vi "gds_usrp_tx.vi"() -> ()   [LabVIEW 2012]
uses:
  <instrlib>/niUSRP/niUSRP Write Tx Data (CDB Cluster).vi
  <vilib>/addons/Modulation/niDMT.lvlib
panel:
  in  "stop":bool
  out "Key Bit Sequence":i8[](array[numeric])
  in  "Plots":enum32{"Constellation", "Transmitted Signal"}(tab)
  out "Constellation Graph":T1(graph) caption="Transmitted Constellation Graph"
  out "Transmitted I Waveform Graph":waveform(dbl)(graph)
  out "Transmitted Q  Waveform Graph":waveform(dbl)(graph)
  out "coerced gain":dbl format="%#_6f"
  out "coerced carrier frequency":dbl=100000.0 format="%#_6p"
  out "coerced IQ rate":dbl=100000.0 format="%#_6p"
  in  "gain":dbl=20.0 format="%#_6f"
  in  "carrier frequency":dbl=433001000.0 format="%#_6p"
  in  "active antenna":string="TX1"
  in  "device names":refnum<k15>="192.168.10.26"
  out "error out":errorcluster
  in  "Modulation Parameters":T2={"TX Parameters"={"Sampling Rate"=1000000.0, "Oversample Factor"=2}, "Shared Parameters"={"Packet Length"=500, "Preamble Length"=20, "modulation type"=enum."OOK", "FSK deviation (Hz)"=625.0, "Filter Parameters"={"modulation type"=enum."ASK", "pulse shaping filter (none)"=enum."none", "filter length (symbols)"=8, "filter parameter"=0.5}}}
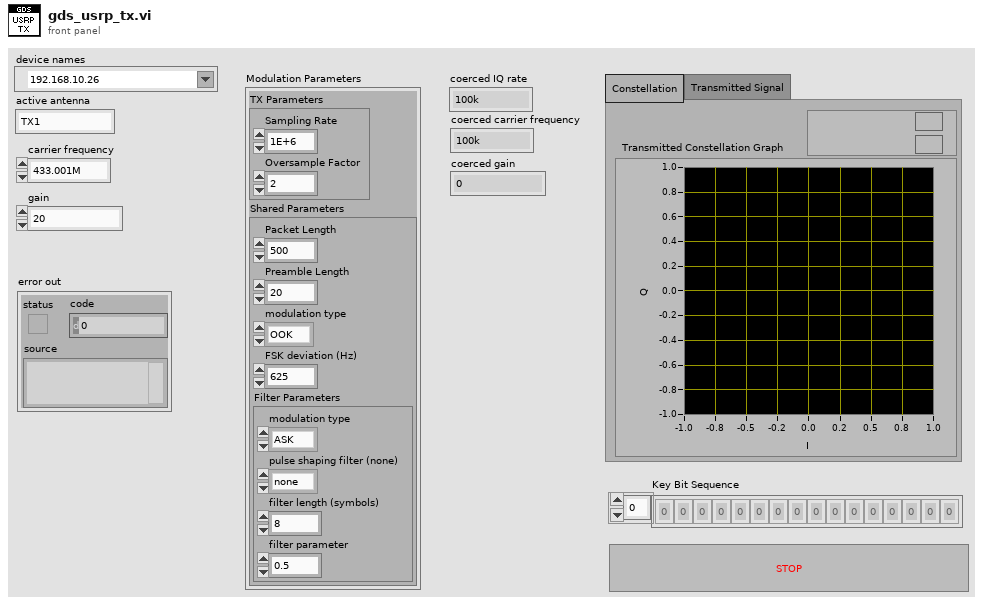
[diagram p1: front panel]
types:
  T1 = cluster{"Decimated Array":dbl[], "Decimated Array":dbl[]}[]
  T2 = cluster{"TX Parameters":cluster{"Sampling Rate":dbl, "Oversample Factor":i32}, "Shared Parameters":cluster{"Packet Length":i32, "Preamble Length":i32, "modulation type":enum16{"OOK", "FSK", "PSK", "QAM", "MSK", "PAM", "ASK", "CPM"}, "FSK deviation (Hz)":dbl, "Filter Parameters":cluster{"modulation type":enum16{"FSK", "PSK", "QAM", "MSK", "PAM", "ASK", "CPM"}, "pulse shaping filter (none)":enum16{"none", "Raised Cosine", "Root Raised Cos", "Gaussian"}, "filter length (symbols)":i32, "filter parameter":dbl}}}
  T3 = typedef "niAMT.lvlib/Complex Data Waveform.ctl" = cluster{"t0":dbl, "dt":dbl, "Y":cdb[]}
  T4 = cluster{"constellation":dbl[], "oversampled data":dbl[]}[]
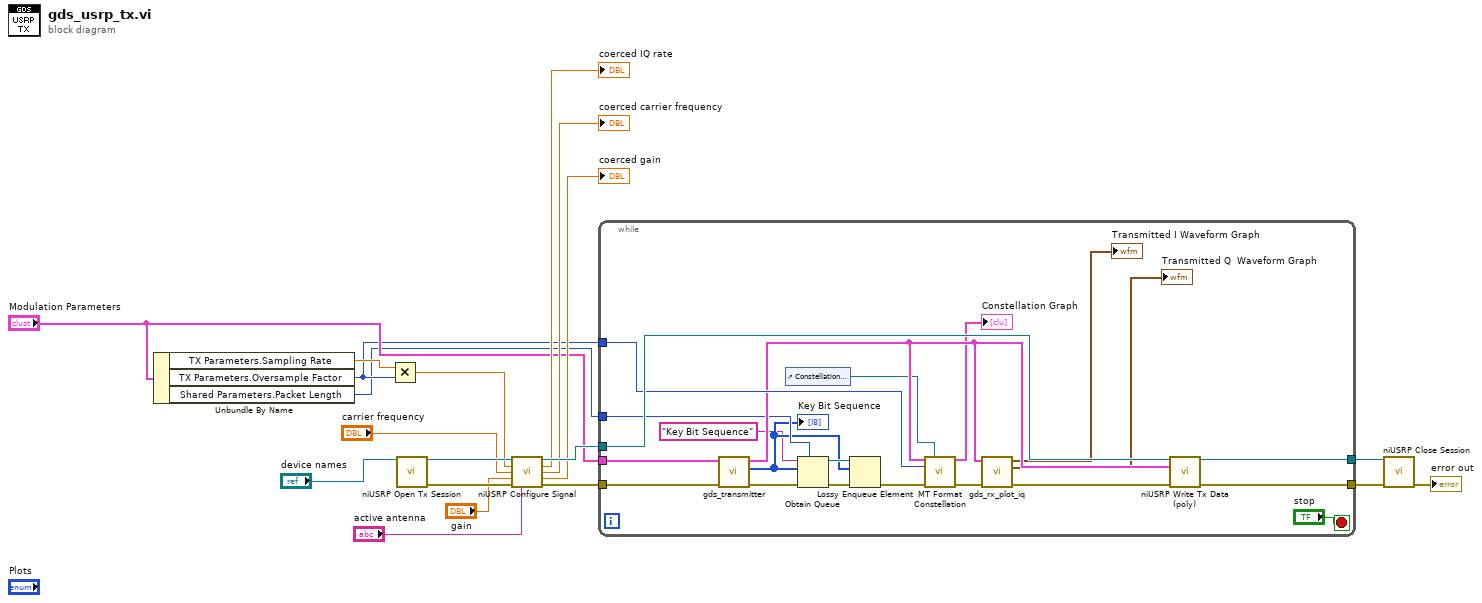
[diagram p0: block diagram]
diagram:
  n1 = Unbundle By Name("Modulation Parameters") -> ("TX Parameters.Sampling Rate"=w4:dbl, "TX Parameters.Oversample Factor"=w2:i32, "Shared Parameters.Packet Length"=w1:i32)
  n2 = Multiply(x=w4, y=w2) -> (x*y=w3:dbl)
  n3 = call <instrlib>:"niUSRP Open Tx Session.vi"("device names"="device names") -> ("session handle out"=w18:refnum<k15>, "error out"=w19:errorcluster)  [unwired: 13 in]
  n4 = call <instrlib>:"niUSRP Configure Signal.vi"("session handle"=w18, "IQ rate"=w3, "carrier frequency"="carrier frequency", "gain"="gain", "error in (no error)"=w19, "active antenna"="active antenna") -> ("session handle out"=w17:refnum<k15>, "coerced IQ rate"=→"coerced IQ rate":dbl, "coerced carrier frequency"=→"coerced carrier frequency":dbl, "coerced gain"=→"coerced gain":dbl, "error out"=w14:errorcluster)  [unwired: 5 in]
  n5 = while {
    tunnel: w17 -> [w40]
    tunnel: [w39] -> w16
    tunnel: [w38] -> w15
    tunnel: w14 -> [w37]
    tunnel: "Modulation Parameters" -> [w36]
    tunnel: w2 -> [w35]
    tunnel: w1 -> [w30]
    stop <- "stop" stop-if-true
    n6 = call "gds_transmitter.vi"("error in (no error)"=w37, "Modulation Parameters"=w36) -> ("error out"=w26:errorcluster, "Key Bit Sequence"=w28:i8[], "Transmitted Signal"=w34:T3)  [unwired: 6 in, 1 out]
    "Key Bit Sequence" <- w28
    n7 = control-ref of="Constellation Graph"() -> (w21:refnum<vi>)
    n8 = Obtain Queue(max queue size (-1, unlimited)=w30, name (unnamed)="Key Bit Sequence", element data type=w28, error in (no error)=w26) -> (queue out=w29:refnum<queue>, error out=w27:errorcluster)  [unwired: 1 in, 1 out]
    n9 = Lossy Enqueue Element(queue=w29, element=w28, error in (no error)=w27) -> (error out=w25:errorcluster)  [unwired: 3 out]
    n10 = call <vilib>:"MT Format Constellation.vi"("waveform"=w34, "constellation reference"=w21, "samples per symbol"=w35, "error in (no error)"=w25) -> ("constellation graph"=→"Constellation Graph":T4, "error out"=w33:errorcluster)  [unwired: 1 in, 9 out]
    n11 = call "gds_rx_plot_iq.vi"("error in"=w33, "Received IQ\nwaveform"=w34) -> ("error out"=w32:errorcluster, "Q component"=→"Transmitted Q  Waveform Graph":waveform(dbl), "I component"=→"Transmitted I Waveform Graph":waveform(dbl))  [unwired: 7 in]
    n12 = call-poly <instrlib>:"niUSRP Write Tx Data (poly).vi"("session handle"=w40, "data"=w34, "error in (no error)"=w32) -> ("session handle out"=w38:refnum<k15>, "error out"=w39:errorcluster)  [unwired: 11 in]
  }
  n13 = call <instrlib>:"niUSRP Close Session.vi"("session handle"=w15, "error in (no error)"=w16) -> ("error out"=→"error out":errorcluster)  [unwired: 13 in]
